vi "hw2p8_hickey.vi"() -> ()   [LabVIEW 2014]
panel:
  out "Required Iterations":i32
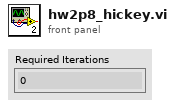
[diagram p1: front panel]
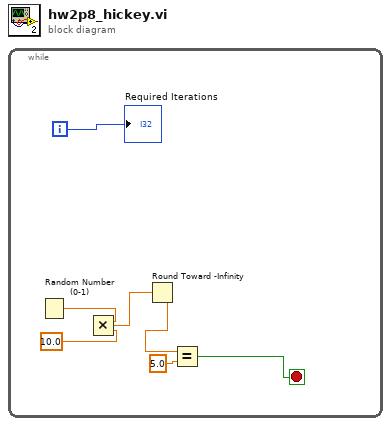
[diagram p0: block diagram]
diagram:
  n1 = while {
    i -> [w4]
    stop <- w3 stop-if-true
    n2 = Random Number (0-1)() -> (number: 0 to 1=w7:dbl)
    n3 = Multiply(x=w7, y=10.0) -> (x*y=w2:dbl)
    n4 = Round Toward -Infinity(1:w2) -> (0:w1:dbl)
    n5 = Equal?(x=w1, y=5.0) -> (x = y?=w3:bool)
    "Required Iterations" <- w4
  }
